vi "RampCTRL_1.vi"(10 "TEMP RAMP":dbl[][](array[numeric]), 11 "Reset 6":bool) -> (1 "Array":dbl[](array[numeric]), 2 "Array 2":dbl[](array[numeric]), 3 "Array 3":dbl[](array[numeric]))   [LabVIEW 2017]
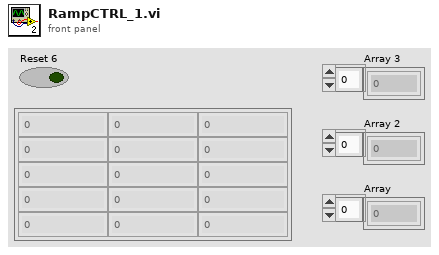
[diagram p1: front panel]
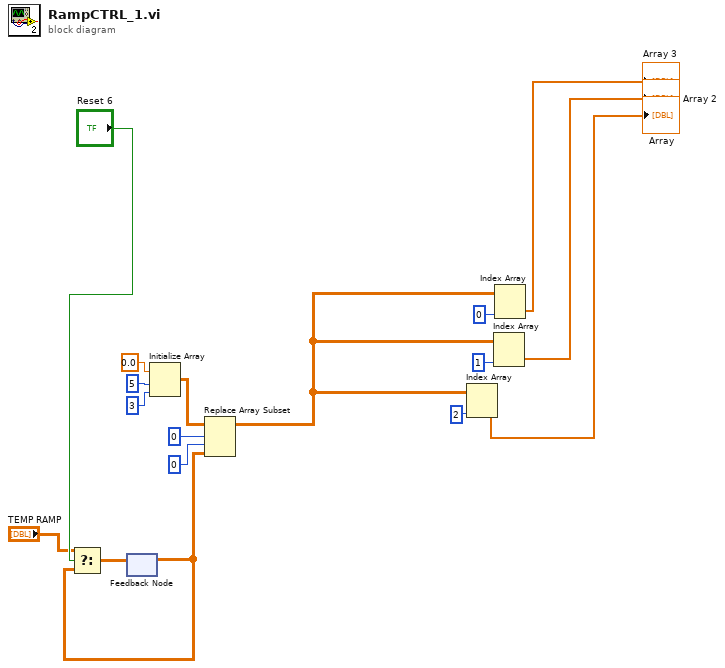
[diagram p0: block diagram]
diagram:
  n1 = feedback #1() -> (w16:dbl[][])  [unwired: 1 in]
  n2 = Select(t="TEMP RAMP", s="Reset 6", f=w16) -> (s? t:f=w15:dbl[][])
  n3 = feedback-in #1(w15) -> ()
  n4 = Initialize Array(0.0 ("element"), 5 ("dimension size"), 3 ("dimension size")) -> (w10:dbl[][])
  n5 = Replace Array Subset(array=w10, new element=w16, index (row)=0, index (col)=0 ("disabled index (col)")) -> (w13:dbl[][])
  n6 = Index Array(array=w13, index (col)=2 ("disabled index (col)")) -> (element=→"Array":dbl[])  [unwired: 1 in]
  n7 = Index Array(array=w13, index (col)=1 ("disabled index (col)")) -> (element=→"Array 2":dbl[])  [unwired: 1 in]
  n8 = Index Array(array=w13, index (col)=0 ("disabled index (col)")) -> (element=→"Array 3":dbl[])  [unwired: 1 in]
